vi "Get SMO HELP.vi"(8 "error in (no error)":errorcluster, 10 "Command":string, 11 "instrument.PPMS in":refnum<class "instrument.PPMS.lvclass">) -> (0 "error out":errorcluster, 2 "help cluster":T1, 3 "instrument.PPMS out":refnum<class "instrument.PPMS.lvclass">)   [LabVIEW 2019, in "instrument.PPMS.lvclass"]
uses:
  instrument.PPMS.lvclass
  <userlib>/LevyLab/Instrument Framework/subsystems/Help/typedefs/Help--cluster.ctl
  <userlib>/LevyLab/Instrument Framework/Instrument Types/Cryostat/Instrument.Cryostat.lvclass
  <userlib>/LevyLab/Instrument Framework/subsystems/Help/Help.lvclass
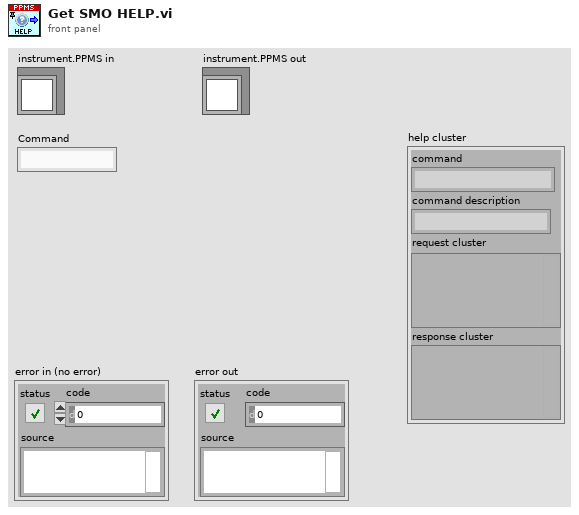
[diagram p1: front panel]
types:
  T1 = typedef "Instrument.lvlib/Help.lvclass/Help--cluster.ctl" = cluster{"command":string, "command description":string, "request cluster":variant, "response cluster":variant}
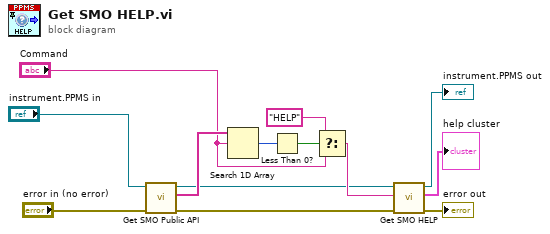
[diagram p0: block diagram]
diagram:
  n1 = call-dynamic "Get SMO Public API.vi"("error in (no error)"="error in (no error)", "instrument.PPMS in"="instrument.PPMS in") -> ("error out"=w2:errorcluster, "Commands"=w7:string[], "instrument.PPMS out"=w4:refnum<class "instrument.PPMS.lvclass">)  [unwired: 7 in]
  n2 = Search 1D Array(1D array=w7, element="Command") -> (index of element=w10:i32)  [unwired: 1 in]
  n3 = Less Than 0?(x=w10) -> (x < 0?=w9:bool)
  n4 = Select(t="HELP", s=w9, f="Command") -> (s? t:f=w6:string)
  n5 = call-parent "Get SMO HELP.vi"("error in (no error)"=w2, "Command"=w6, "Instrument.Cryostat in"=w4) -> ("error out"=→"error out":errorcluster, "help cluster"=→"help cluster":T1, "Instrument.Cryostat out"=→"instrument.PPMS out":refnum<class "instrument.PPMS.lvclass">)  [unwired: 6 in]
